vi "Supported Smart Syntax Representation.vi"(0 "Message Popup in":refnum<class "ControllerData.lvclass">, 11 "error in (no error)":errorcluster) -> (4 "Message Popup out":refnum<class "ControllerData.lvclass">, 6 "Smart Syntax Representation List":string[](array[string]), 15 "error out":errorcluster)   [LabVIEW 2019, in "ControllerData.lvclass"]
uses:
  ControllerData.lvclass
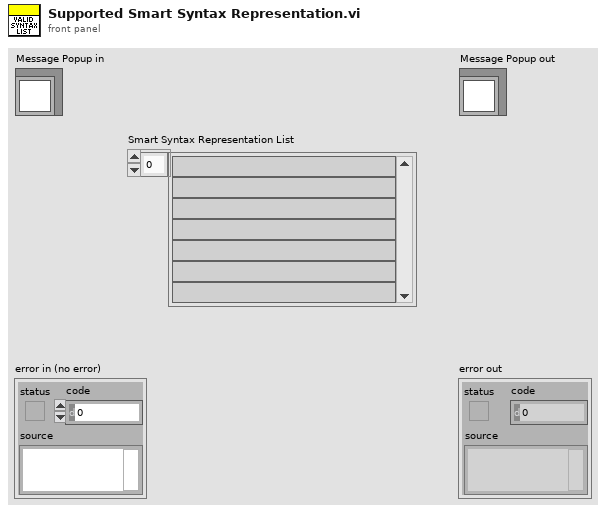
[diagram p1: front panel]
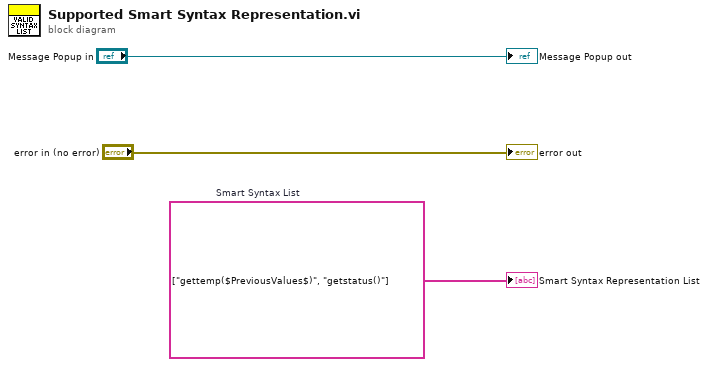
[diagram p0: block diagram]
diagram:
  w1 = string[] ["gettemp($PreviousValues$)", "getstatus()"]  # Smart Syntax List
  "error out" <- "error in (no error)"
  "Message Popup out" <- "Message Popup in"
  "Smart Syntax Representation List" <- w1
